vi "PH_Class.destructor.vi"(0 "i ref in":refnum<vi>, 5 "error in(no error)":errorcluster) -> (19 "error out":errorcluster)   [LabVIEW 2014, in "PH_Class.lvlib"]
doc: "This is the destructor of a class.\n\nLicense Agreement for this software:\n\nCopyright (C)\nGesellschaft für Schwerionenforschung, GSI\nPlanckstr. 1\n64291 Darmstadt\nGermany\n\nContact: D.Beck@gsi.de \n\nThis program is free software; you can redistribute it and/or modify it under the terms of the \nGNU General Public License as published by the Free Software Foundation; either version 2 of \nthe license, or (at your option) any later version.\n\nThis program is distributed in the hope that it will be useful, but WITHOUT ANY WARRANTY; \nwithout even the implied warranty of MERCHANTABILITY or FITNESS FOR A PARTICULAR PURPOSE. See the GNU General License for more details (http://www.gnu.org).\n\nGesellschaft für Schwerionenforschung, GSI\nPlanckstr. 1, 64291 Darmstadt, Germany\nFor all questions and ideas contact: M.Richter@gsi.de, H.Brand@gsi.de or D.Beck@gsi.de.\nLast update: 16-JUN-2004"
uses:
  PH_Class.lvlib
  CSCore/BaseGUI/BaseGUI.lvlib
  PH_Common/PH_Common.lvlib
  CSCore/BaseProcess/BaseProcess.lvlib
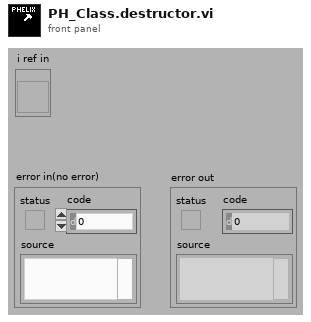
[diagram p1: front panel]
types:
  T1 = typedef "PH_Class.lvlib/PH_Class.i attribute.ctl" = cluster{"Event":refnum<user-event>, "Event registered":refnum<k4>, "GUI Refs stored":refnum<k4>}
  T2 = enum16{"SetAttribute", "GetAttribute", "CreateAttribute", "DestroyAttribute", "DestroyAllAtributes"}
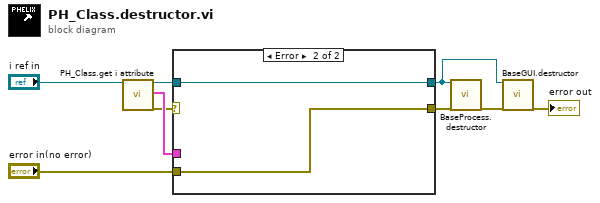
[diagram p0: block diagram]
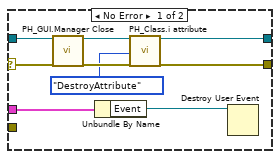
[diagram p2: hidden frame]
diagram:
  n1 = call "PH_Class.get i attribute.vi"("i ref in"="i ref in") -> ("i ref out"=w4:refnum<vi>, "i attribute"=w3:T1, "error out"=w2:errorcluster)  [unwired: 16 in]
  n2 = case shown="Error" w2 {
    selector: w2 -> [w10 _]
    tunnel: [w14 w20] -> w7
    tunnel: [w16 w19] -> w6
    tunnel: w4 -> [w17 w20]
    tunnel: w3 -> [w12 _]
    tunnel: "error in(no error)" -> [_ w19]
    frame No Error {
      n3 = call "PH_GUI.Manager Close.vi"("i ref in"=w17, "error in"=w10) -> ("i ref out"=w15:refnum<vi>, "error out"=w18:errorcluster)  [unwired: 16 in]
      n4 = Unbundle By Name(w12) -> ("Event"=w11:refnum<user-event>)
      n5 = call "PH_Class.i attribute.vi"("VI Refnum"=w15, "Action"=T2."DestroyAttribute", "error in (no error)"=w18) -> ("VI Refnum out"=w14:refnum<vi>, "error out"=w16:errorcluster)  [unwired: 14 in, 1 out]
      n6 = Destroy User Event(user event=w11) -> ()  [unwired: 1 in, 1 out]
    }
    frame Error {
    }
  }
  n7 = call "BaseProcess.destructor.vi"("i ref in"=w7, "error in (no error)"=w6) -> ("error out"=w9:errorcluster)  [unwired: 17 in]
  n8 = call "BaseGUI.destructor.vi"("i ref in"=w7, "error in (no error)"=w9) -> ("error out"=→"error out":errorcluster)  [unwired: 17 in]
